vi "test_Create FPGA Addon--Error.vi"(8 "error in (no error)":errorcluster, 11 "TestCase in":refnum<class "Scripting API Unit Tests.lvclass">) -> (0 "error out":errorcluster, 3 "TestCase out":refnum<class "Scripting API Unit Tests.lvclass">)   [LabVIEW 2018, in "Scripting API Unit Tests.lvclass"]
uses:
  Scripting API Unit Tests.lvclass
  <vilib>/addons/_JKI Toolkits/VI Tester/TestCase.llb/TestCase.lvclass
  FPGA Addon Test Class/FPGA Addon Test Class.lvclass
  APIs/Scripting API/Scripting API.lvlib
  C:/Program Files (x86)/National Instruments/LabVIEW 2018/vi.lib/addons/_JKI Toolkits/VI Tester/TestCase.llb/TestCase.lvclass
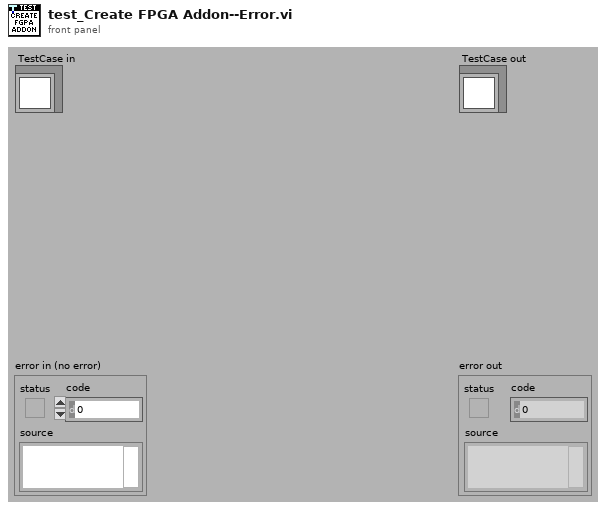
[diagram p1: front panel]
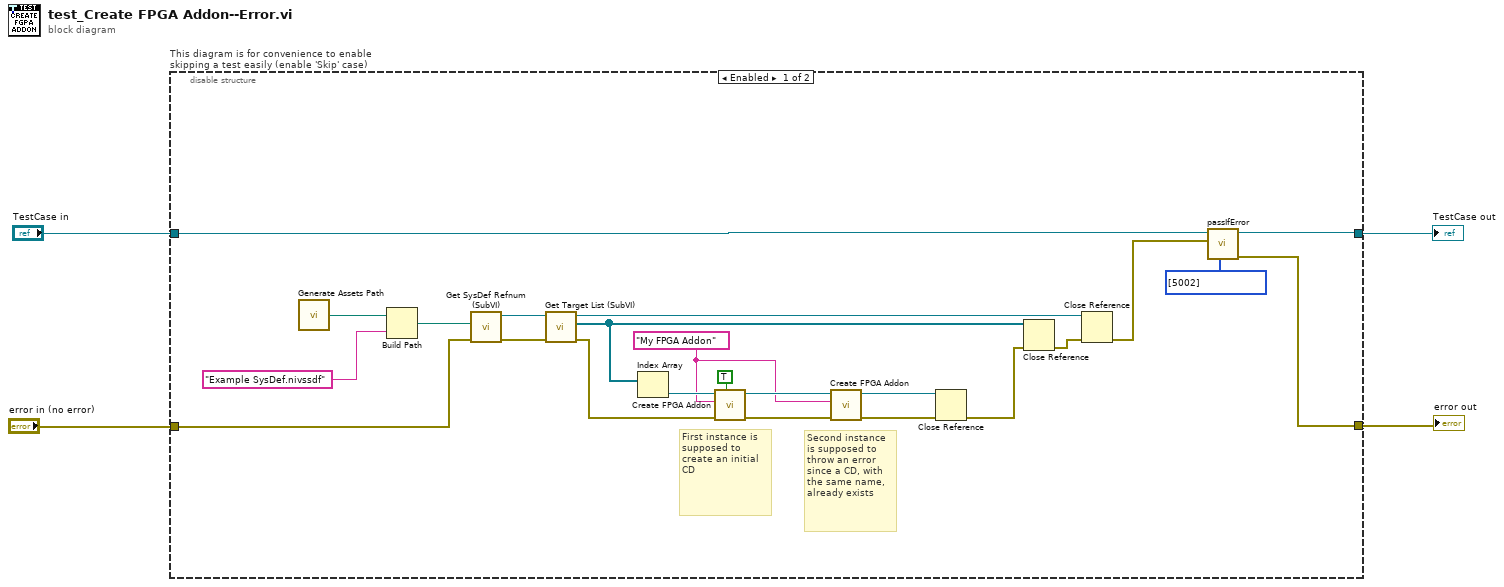
[diagram p0: block diagram]
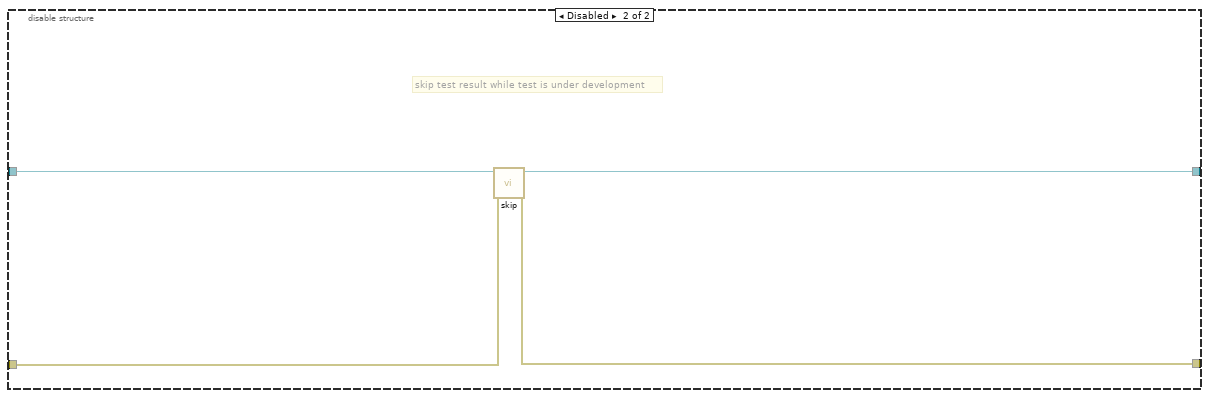
[diagram p2: hidden frame]
diagram:
  n1 = disable-structure "This diagram is for convenience to enable skipping a test easily (enable 'Skip' case)" shown="Enabled" {
    disable-tunnel: "TestCase in" -> [w9 w31]
    disable-tunnel: [w7 w29] -> w1
    disable-tunnel: [w6 w30] -> w3
    disable-tunnel: "error in (no error)" -> [w22 w28]
    frame Enabled {
      w13 = "My FPGA Addon" ("FPGA addon name")
      # "Second instance is supposed to throw an error since a CD, with the same name, already exists"
      # "First instance is supposed to create an initial CD"
      n2 = call "Generate Assets Path.vi"() -> ("Assets path"=w27:path)
      n3 = Build Path(base path=w27, name or relative path="Example SysDef.nivssdf") -> (appended path=w25:path)
      n4 = call "Get SysDef Refnum (SubVI).vi"("error in (no error)"=w22, "System Definition path"=w25) -> ("error out"=w21:errorcluster, "SysDef Refnum out"=w24:refnum<k24>)  [unwired: 8 in]
      n5 = call "Get Target List (SubVI).vi"("error in (no error)"=w21, "SysDef Refnum in"=w24) -> ("error out"=w20:errorcluster, "Target List Refnums"=w19:refnum<k24>[], "SysDef Refnum out"=w18:refnum<k24>)  [unwired: 7 in]
      n6 = Index Array(array=w19) -> (element=w23:refnum<k24>)  [unwired: 1 in]
      n7 = call "Create FPGA Addon.vi"("group scalars"=TRUE, "error in"=w20, "FPGA addon name"=w13, "target in"=w23) -> ("error out"=w15:errorcluster, "target out"=w14:refnum<k24>)  [unwired: 5 in, 1 out]
      n8 = call "Create FPGA Addon.vi"("error in"=w15, "FPGA addon name"=w13, "target in"=w14) -> ("error out"=w11:errorcluster, "target out"=w12:refnum<k24>)  [unwired: 6 in, 1 out]
      n9 = Close Reference(reference=w12, error in (no error)=w11) -> (error out=w10:errorcluster)
      n10 = Close Reference(reference=w19, error in (no error)=w10) -> (error out=w17:errorcluster)
      n11 = Close Reference(reference=w18, error in (no error)=w17) -> (error out=w5:errorcluster)
      n12 = call-dynamic "passIfError.vi"("passing error codes (default = any error code)"=i32[] [5002], "error"=w5, "TestCase in"=w9) -> ("error out"=w6:errorcluster, "TestCase out"=w7:refnum<class "Scripting API Unit Tests.lvclass">)  [unwired: 7 in]
    }
    frame Disabled {
      # "skip test result while test is under development"
      n13 = call <vilib>:"skip.vi"("error in (no error)"=w28, "TestCase in"=w31) -> ("error out"=w30:errorcluster, "TestCase out"=w29:refnum<class "Scripting API Unit Tests.lvclass">)  [unwired: 8 in]
    }
  }
  "error out" <- w3
  "TestCase out" <- w1
